vi "闹钟（小时）.vi"(5 "设置小时":i32=5, 7 "启用":bool=TRUE) -> (6 "时间到脉冲":bool, 8 "小时":i32)   [LabVIEW 2012]
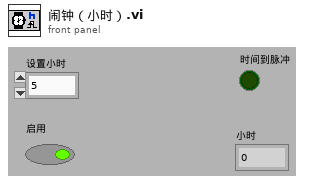
[diagram p1: front panel]
types:
  T1 = typedef "LVDateTimeRec.ctl" = cluster{"秒数的小数部分":dbl, "秒":i32, "分":i32, "时":i32, "日":i32, "月":i32, "年":i32, "天数（周）":i32, "天数（年）":i32, "DST":i32}
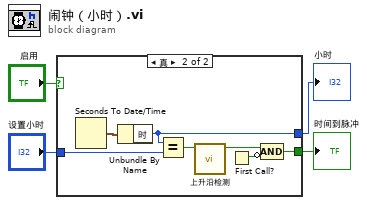
[diagram p0: block diagram]
diagram:
  n1 = case shown="真" "启用" {
    tunnel: "设置小时" -> [_ w6]
    tunnel: [_ w10] -> w2
    tunnel: [_ w7] -> w1
    frame False {
    }
    frame True {
      n2 = Seconds To Date/Time() -> (date time rec=w11:T1)  [unwired: 2 in]
      n3 = Unbundle By Name(w11) -> ("时"=w7:i32)
      n4 = Equal?(x=w7, y=w6) -> (x = y?=w8:bool)
      n5 = call "上升沿检测.vi"("input"=w8) -> ("output"=w5:bool)  [unwired: 9 in, 1 out]
      n6 = First Call?() -> (First Call?: T/F=w9:bool)
      n7 = Compound Arithmetic op=AND(w5, invert w9) -> (w10:bool)
    }
  }
  "时间到脉冲" <- w2
  "小时" <- w1
